vi "v4.0.vi"() -> ()   [LabVIEW 2018]
uses:
  <vilib>/DAQmx/read.llb/DAQmx Read (Analog 1D DBL NChan 1Samp).vi
  <extravilib>/ChannelInstances/High Speed Stream-c(a[.](c(dbl,dbl,dbl,dbl)),stamp,a[.](dbl),c(dbl,dbl,dbl,dbl,dbl,dbl,dbl))/_Read For Replicate.vi
  <extravilib>/ChannelInstances/High Speed Stream-c(a[.](c(dbl,dbl,dbl,dbl)),stamp,a[.](dbl),c(dbl,dbl,dbl,dbl,dbl,dbl,dbl))/Instantiate.vi
  <extravilib>/ChannelInstances/High Speed Stream-c(a[.](c(dbl,dbl,dbl,dbl)),stamp,a[.](dbl),c(dbl,dbl,dbl,dbl,dbl,dbl,dbl))/)Channel.vi
  <extravilib>/ChannelInstances/High Speed Stream-c(a[.](c(dbl,dbl,dbl,dbl)),stamp,a[.](dbl),c(dbl,dbl,dbl,dbl,dbl,dbl,dbl))/Abort Signal/Init Signal.vi
  <vilib>/Utility/file.llb/Write Delimited Spreadsheet (string).vi
  <vilib>/DAQmx/create/channels.llb/DAQmx Create Channel (AI-Temperature-Thermocouple).vi
  <vilib>/DAQmx/configure/timing.llb/DAQmx Timing (Sample Clock).vi
  <vilib>/DAQmx/miscellaneous.llb/DAQmx Fill In Error Info.vi
  <extravilib>/ChannelInstances/High Speed Stream-c(a[.](c(dbl,dbl,dbl,dbl)),stamp,a[.](dbl),c(dbl,dbl,dbl,dbl,dbl,dbl,dbl)).lvlib
  <resource>/objmgr/daqmx.rc
panel:
  out "SampClk.Rate":dbl
  out "Current Time":timestamp
  out "DAQmx Data":T1
  out "Rig Temperatures":T2
  out "Flowrate Data":T3(array[cluster])
  out "UI Current Time":timestamp format="%<%X\n%x>T"
  out "DAQ Current Time":timestamp format="%<%X\n%x>T"
  in  "file path (dialog if empty)":path
  out "Enum":T4(ring)
  in  "Start Recording?":bool
  in  "Stop Recording?":bool
  in  "Flowrate Control":dbl
  out "Status":T5(ring)
  in  "OK Button":bool
  in  "DAQ Properties":cluster{"Sample Rate [Hz]":dbl}={"Sample Rate [Hz]"=1.0} {"Sample Rate [Hz]" min=0.1 max=10000.0 step=0.1}
  # "Line Data [ °C]"
  # "Rig Temperatures [ °C]"
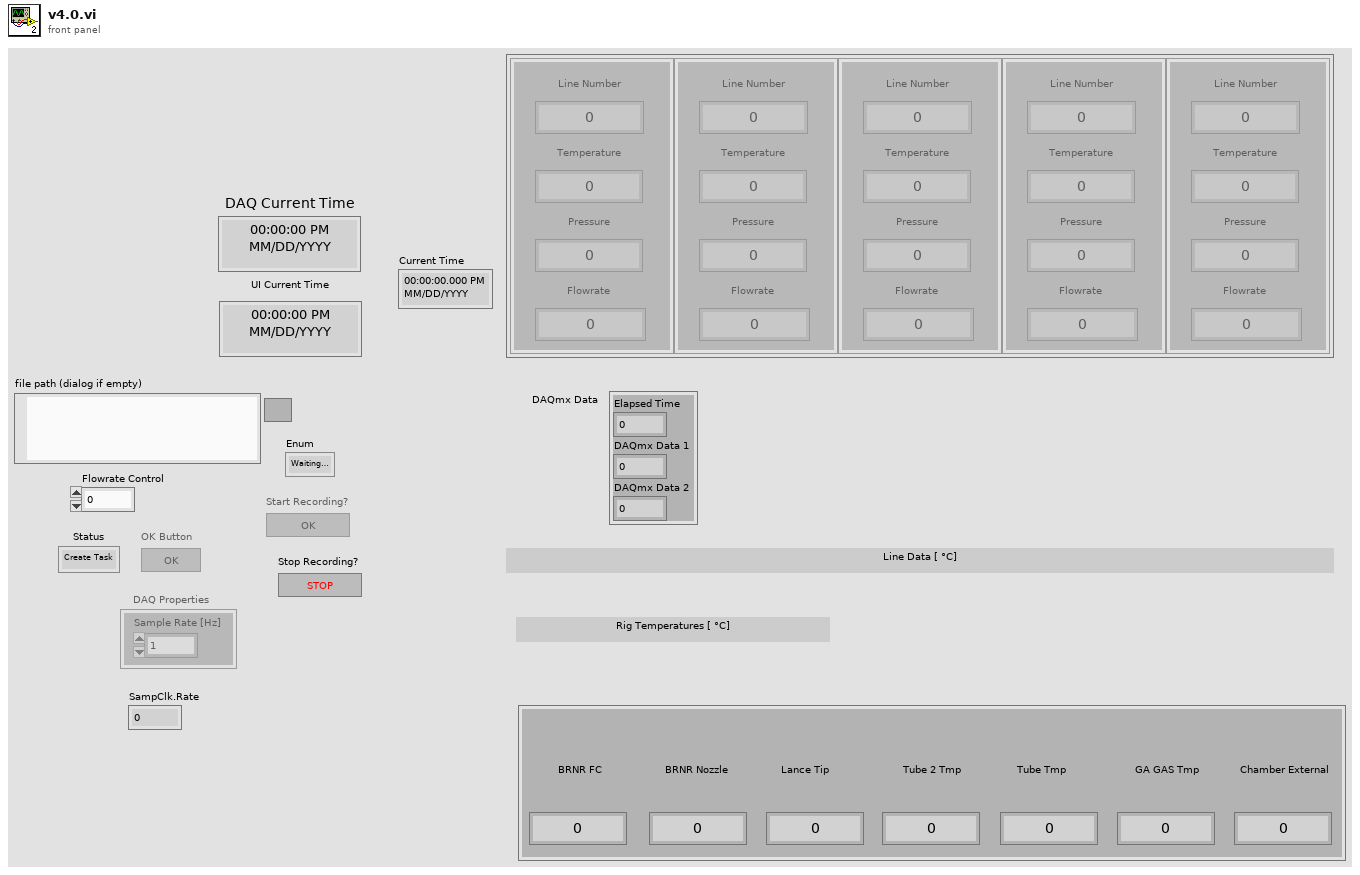
[diagram p1: front panel]
types:
  T1 = cluster{"Elapsed Time":dbl, "DAQmx Data 1":dbl, "DAQmx Data 2":dbl}
  T2 = cluster{"BRNR FC":dbl, "BRNR Nozzle":dbl, "Lance Tip":dbl, "Tube 2 Tmp":dbl, "Tube Tmp":dbl, "GA GAS Tmp":dbl, "Chamber External":dbl}
  T3 = cluster{"Line Number":dbl, "Temperature":dbl, "Pressure":dbl, "Flowrate":dbl}[]
  T4 = enum16{"Waiting to record", "Creating Spreadsheet", "Recording", "Finished Recording"}
  T5 = enum16{"Create Task", "Change Settings", "Check Settings", "Read Data", "End Task"}
  T6 = enum8{"Enabled", "Disabled", "Disabled and Grayed Out"}
  T7 = cluster{"Flowrate Data":cluster{"Line Number":dbl, "Temperature":dbl, "Pressure":dbl, "Flowrate":dbl}[], "Current Time":timestamp, "DAQmx Data":dbl[], "Rig Temperatures":cluster{"BRNR FC":dbl, "BRNR Nozzle":dbl, "Lance Tip":dbl, "Tube 2 Tmp":dbl, "Tube Tmp":dbl, "GA GAS Tmp":dbl, "Chamber External Temp":dbl}}
  T8 = cluster{"BRNR FC":dbl, "BRNR Nozzle":dbl, "Lance Tip":dbl, "Tube 2 Tmp":dbl, "Tube Tmp":dbl, "GA GAS Tmp":dbl, "Chamber External Temp":dbl}
  T9 = typedef "High Speed Stream-c(a[.](c(dbl,dbl,dbl,dbl)),stamp,a[.](dbl),c(dbl,dbl,dbl,dbl,dbl,dbl,dbl)).lvlib/)Channel.ctl" = refnum<queue>
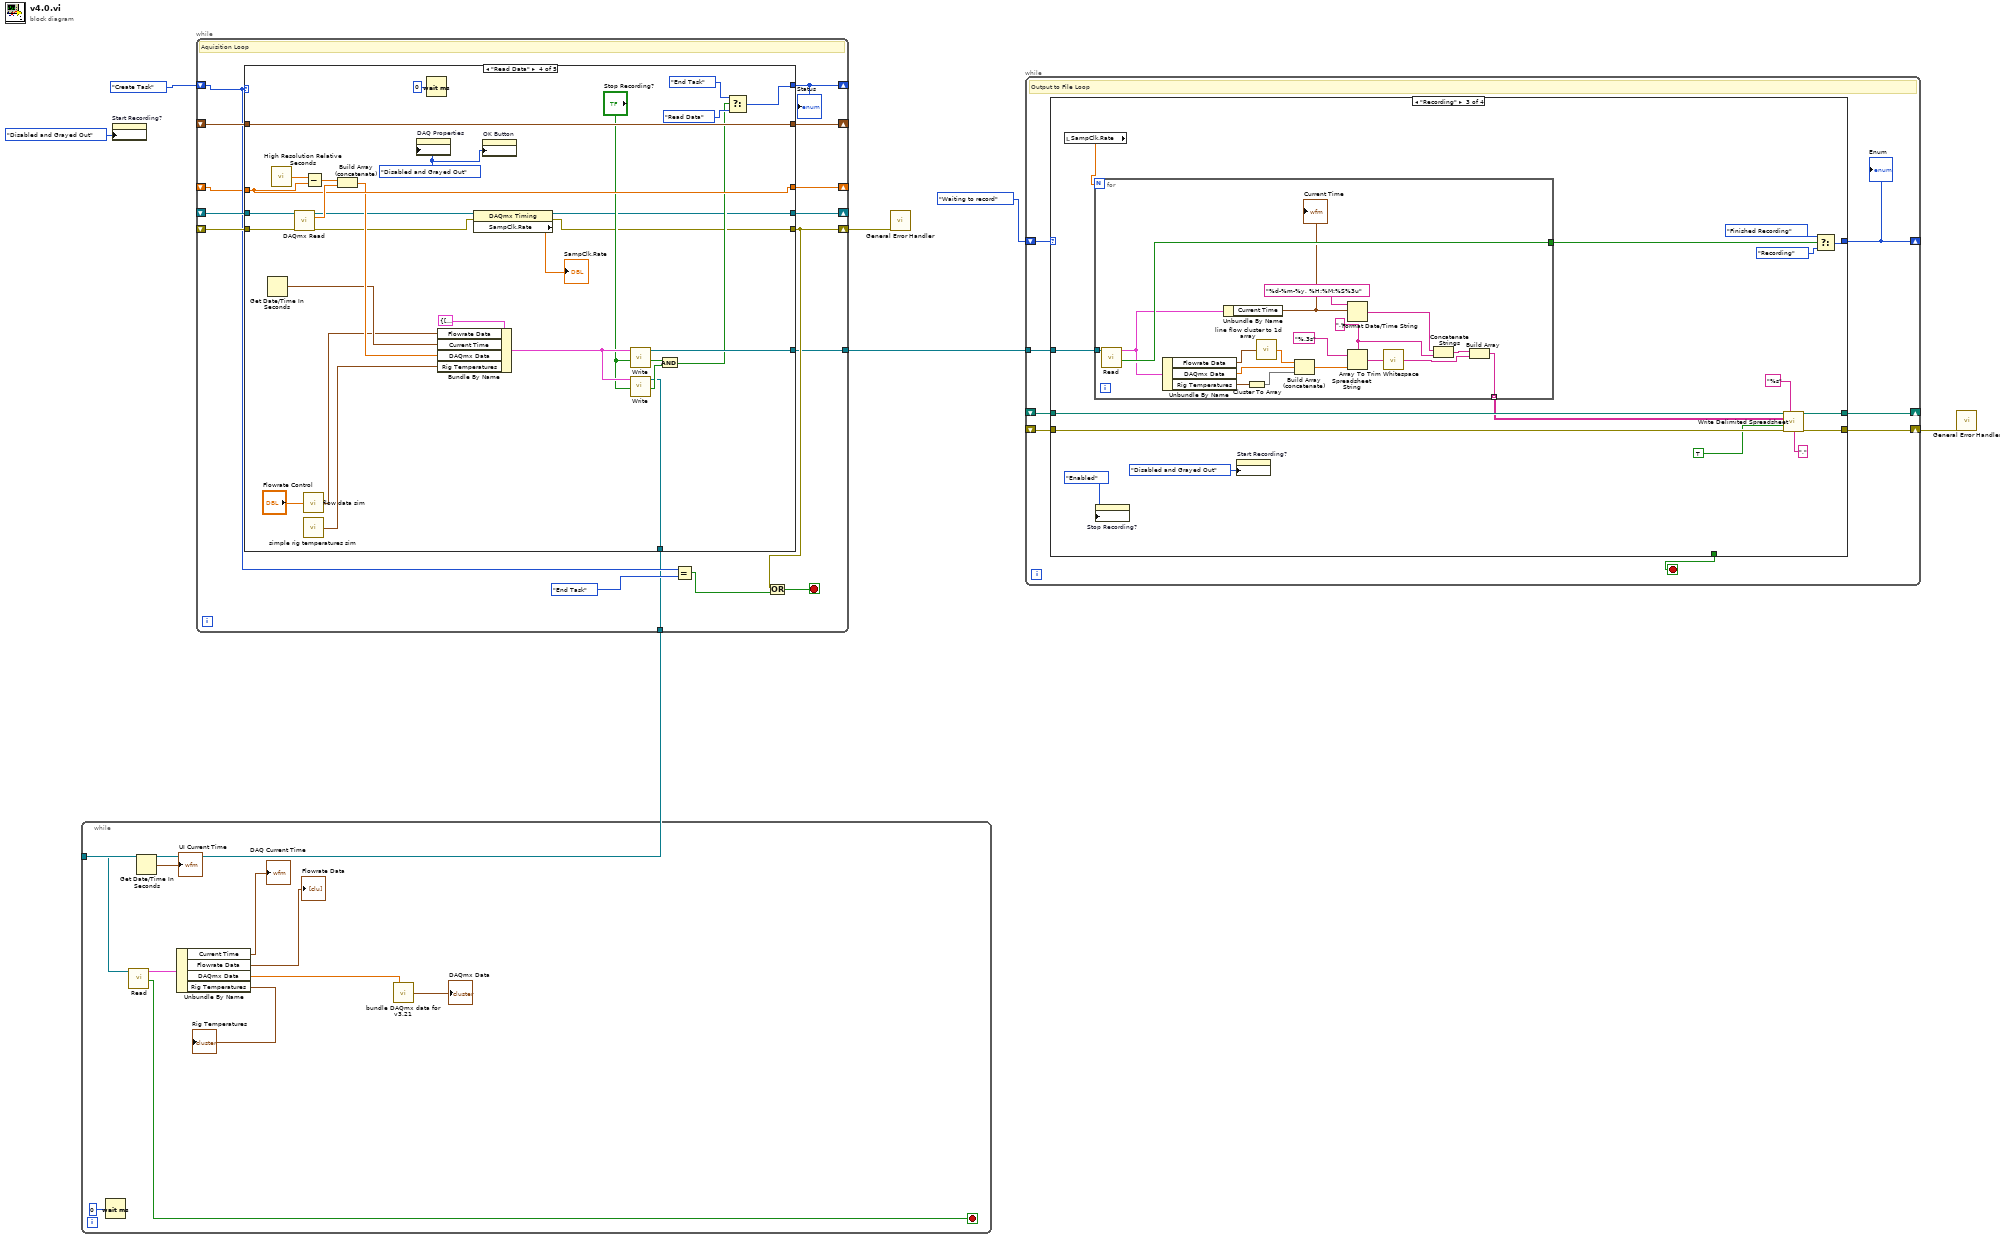
[diagram p0: block diagram]
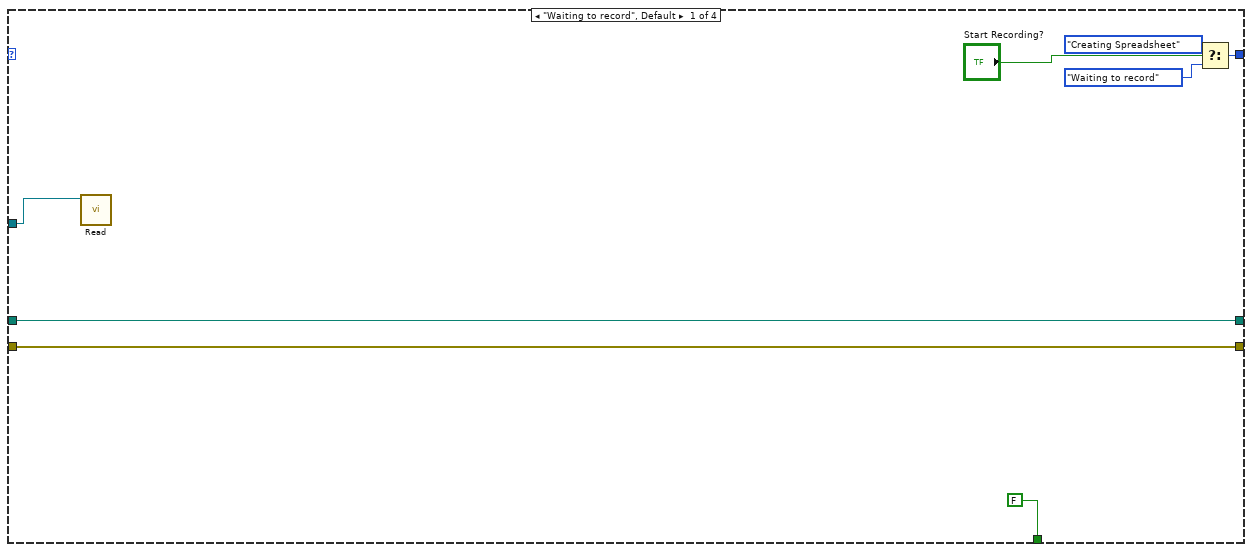
[diagram p2: hidden frame]
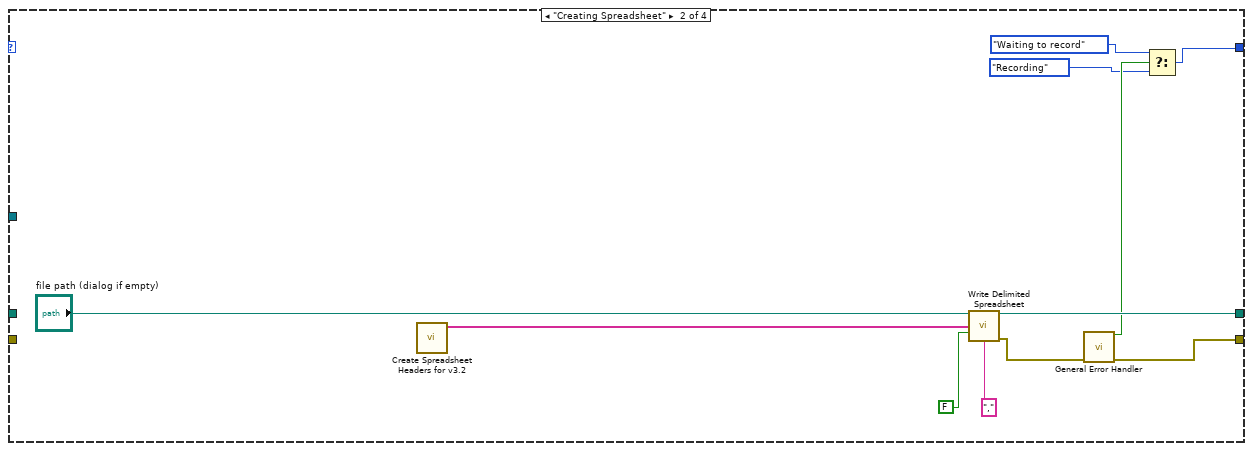
[diagram p3: hidden frame]
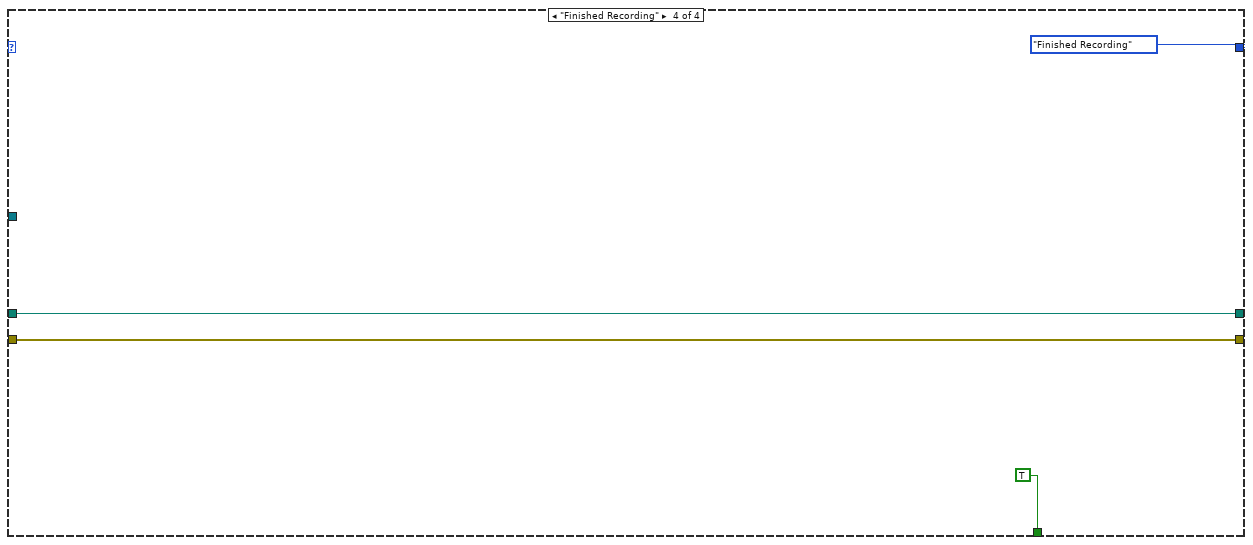
[diagram p4: hidden frame]
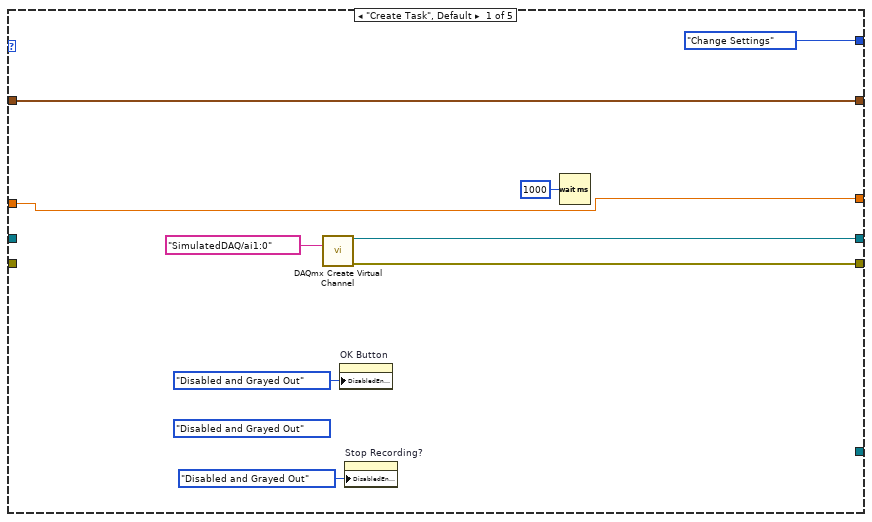
[diagram p5: hidden frame]
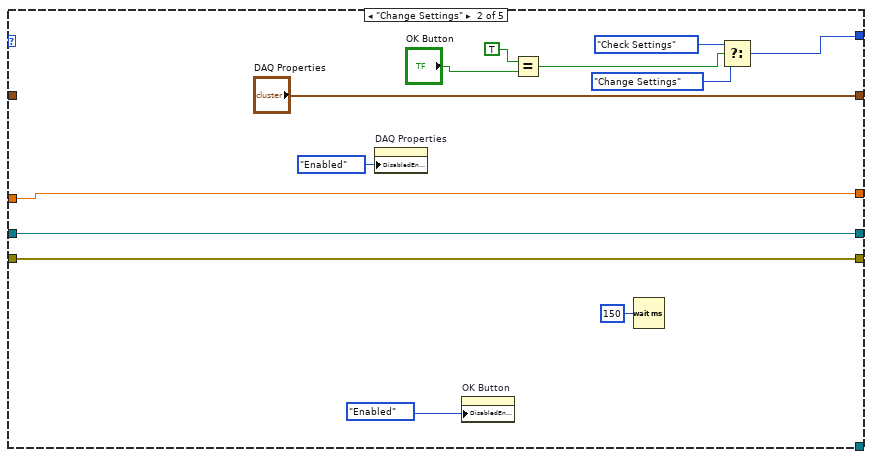
[diagram p6: hidden frame]
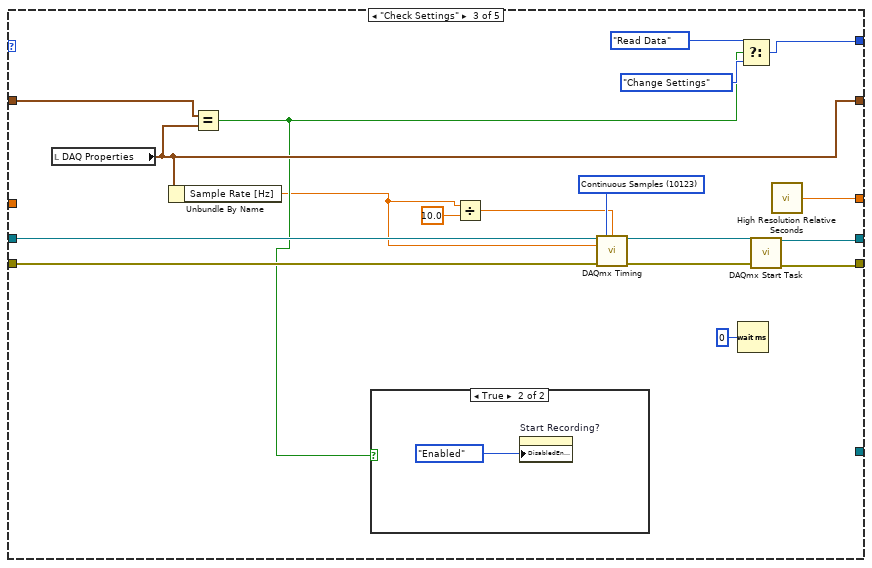
[diagram p7: hidden frame]
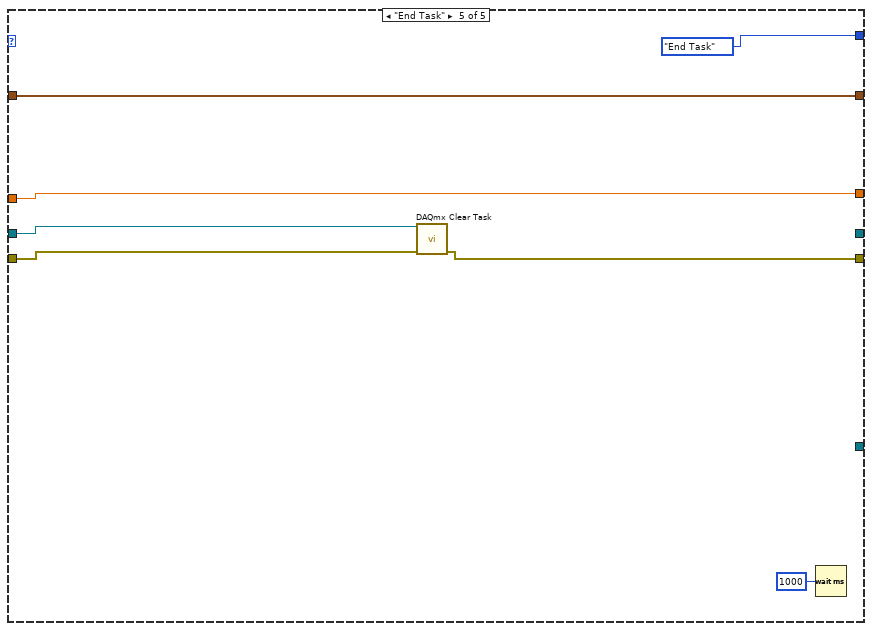
[diagram p9: hidden frame]
diagram:
  n1 = property on="Start Recording?" class="Bool"("DisabledEnum"=T6."Disabled and Grayed Out" ("Disabled")) -> ()  [unwired: 2 in, 2 out]
  n2 = while {
    shift-right: [w17] -> _
    shift-left: T5."Create Task" -> [w13]
    shift-right: [w22] -> _
    shift-left: _ -> [w20]
    shift-right: [w16] -> w3
    shift-left: _ -> [w19]
    shift-right: [w21] -> _
    shift-left: _ -> [w18]
    shift-right: [w12] -> _
    shift-left: _ -> [w11]
    tunnel: [w9] -> w5
    tunnel: [w8] -> w1
    stop <- w10 stop-if-true
    # "Aquisition Loop"
    n3 = case shown="\"Read Data\"" w13 {
      tunnel: [w31 w44 w52 w66 _] -> w22
      tunnel: [w30 w43 w51 w67 w100] -> w16
      tunnel: [T5."Change Settings" w37 w58 w89 T5."End Task"] -> w17
      tunnel: [w27 "DAQ Properties" w55 w91 w99] -> w21
      tunnel: w20 -> [_ w44 w57 w93 w97]
      tunnel: w19 -> [_ w43 w56 w92 w96]
      tunnel: w18 -> [w27 _ w62 w91 w99]
      tunnel: [w25 w34 w49 w83 w95] -> w12
      tunnel: w11 -> [w25 w34 _ w83 w95]
      tunnel: [_ _ _ w76 _] -> w9
      tunnel: [_ _ _ w69 _] -> w8
      frame "Create Task", Default {
        (unwired) T6."Disabled and Grayed Out" ("Disabled")
        n4 = call-poly <vilib>:"DAQmx Create Virtual Channel.vi"("physical channels"=tag "SimulatedDAQ/ai1:0") -> ("task out"=w31:refnum<k21>, "error out"=w30:errorcluster)  [unwired: 13 in]
        n5 = property on="OK Button" class="Bool"("DisabledEnum"=T6."Disabled and Grayed Out" ("Disabled")) -> ()  [unwired: 2 in, 2 out]
        n6 = property on="Stop Recording?" class="Bool"("DisabledEnum"=T6."Disabled and Grayed Out" ("Disabled")) -> ()  [unwired: 2 in, 2 out]
        n7 = Wait (ms)(milliseconds to wait=u32 1000) -> ()  [unwired: 1 out]
      }
      frame "Change Settings" {
        n8 = property on="DAQ Properties" class="Clust (strict)"("DisabledEnum"=T6."Enabled" ("Disabled")) -> ()  [unwired: 2 in, 2 out]
        n9 = property on="OK Button" class="Bool"("DisabledEnum"=T6."Enabled" ("Disabled")) -> ()  [unwired: 2 in, 2 out]
        n10 = Equal?(x=TRUE, y="OK Button") -> (x = y?=w39:bool)
        n11 = Wait (ms)(milliseconds to wait=u32 150) -> ()  [unwired: 1 out]
        n12 = Select(t=T5."Check Settings", s=w39, f=T5."Change Settings") -> (s? t:f=w37:T5)
      }
      frame "Check Settings" {
        w50 = 10123 items=["Finite Samples"=10178, "Continuous Samples"=10123, "Hardware Timed Single Point"=12522] ("sample mode")
        n13 = local read "DAQ Properties"() -> (w55:cluster{"Sample Rate [Hz]":dbl})
        n14 = Unbundle By Name(w55) -> ("Sample Rate [Hz]"=w46:dbl)
        n15 = Equal?(x=w62, y=w55) -> (x = y?=w48:bool)
        n16 = case shown="True" w48 {
          frame False {
          }
          frame True {
            n17 = property on="Start Recording?" class="Bool"("DisabledEnum"=T6."Enabled" ("Disabled")) -> ()  [unwired: 2 in, 2 out]
          }
        }
        n18 = Divide(x=w46, y=10.0) -> (x/y=w45:dbl)
        n19 = call-poly <vilib>:"DAQmx Timing.vi"("task/channels in"=w57, "sample mode"=w50, "samples per channel"=w45, "rate"=w46, "error in"=w56) -> ("task out"=w54:refnum<k21>, "error out"=w53:errorcluster)  [unwired: 9 in]
        n20 = Wait (ms)(milliseconds to wait=u32 0) -> ()  [unwired: 1 out]
        n21 = Select(t=T5."Read Data", s=w48, f=T5."Change Settings") -> (s? t:f=w58:T5)
        n22 = call <vilib>:"DAQmx Start Task.vi"("task/channels in"=w54, "error in"=w53) -> ("task out"=w52:refnum<k21>, "error out"=w51:errorcluster)  [unwired: 12 in]
        n23 = call <vilib>:"High Resolution Relative Seconds.vi"() -> ("relative seconds"=w49:dbl)
      }
      frame "Read Data" {
        w75 = T6."Disabled and Grayed Out" ("Disabled")
        n24 = Get Date/Time In Seconds() -> (seconds since 1Jan1904=w79:timestamp)
        n25 = call <vilib>:"High Resolution Relative Seconds.vi"() -> ("relative seconds"=w86:dbl)
        n26 = call-poly <vilib>:"DAQmx Read.vi"("task/channels in"=w93, "error in"=w92) -> ("task out"=w68:refnum<k21>, "data"=w85:dbl[], "error out"=w65:errorcluster)  [unwired: 11 in]
        n27 = call "simple rig temperatures sim.vi"() -> ("Rig Temperatures"=w77:T8)
        n28 = call "flow data sim.vi"("Offset"="Flowrate Control") -> ("Flowrate Data"=w78:T3)
        n29 = Subtract(x=w86, y=w83) -> (x-y=w84:dbl)
        n30 = Build Array (concatenate)(w84, w85) -> (w80:dbl[])
        n31 = property on="DAQ Properties" class="Clust (strict)"("DisabledEnum"=w75) -> ()  [unwired: 2 in, 2 out]
        n32 = Wait (ms)(milliseconds to wait=u32 0) -> ()  [unwired: 1 out]
        n33 = Bundle By Name(cluster=T7 {"Flowrate Data"=[{"Line Number"=1.0, "Temperature"=17.480721541683437, "Pressure"=24.0, "Flowrate"=0.0}, {"Line Number"=2.0, "Temperature"=21.850901927104296, "Pressure"=30.0, "Flowrate"=0.0}, {"Line Number"=3.0, "Temperature"=26.221082312525155, "Pressure"=36.0, "Flowrate"=0.0}, {"Line Number"=4.0, "Temperature"=30.591262697946018, "Pressure"=42.00000000000001, "Flowrate"=0.0}, {"Line Number"=5.0, "Temperature"=34.96144308336687, "Pressure"=48.0, "Flowrate"=0.0}], "Current Time"=timestamp(0 s since 1904-01-01), "DAQmx Data"=[], "Rig Temperatures"={"BRNR FC"=0.0, "BRNR Nozzle"=0.0, "Lance Tip"=0.0, "Tube 2 Tmp"=0.0, "Tube Tmp"=0.0, "GA GAS Tmp"=0.0, "Chamber External Temp"=0.0}}, "Flowrate Data"=w78, "Current Time"=w79, "DAQmx Data"=w80, "Rig Temperatures"=w77) -> (w74:T7)
        n34 = property class="DAQmx Timing"(reference=w68, error in=w65) -> (reference out=w66:refnum<k21>, error out=w67:errorcluster, "SampClk.Rate"=→"SampClk.Rate":dbl)
        n35 = property on="OK Button" class="Bool"("DisabledEnum"=w75) -> ()  [unwired: 2 in, 2 out]
        n36 = call <extravilib>:"Write.vi"("last element? (F)"="Stop Recording?", "element"=w74) -> ("done?"=w72:bool, "channel"=w76:T9)  [unwired: 7 in, 1 out]
        n37 = call <extravilib>:"Write.vi"("last element? (F)"="Stop Recording?", "element"=w74) -> ("done?"=w71:bool, "channel"=w69:T9)  [unwired: 7 in, 1 out]
        n38 = And(x=w72, y=w71) -> (x .and. y?=w70:bool)
        n39 = Select(t=T5."End Task", s=w70, f=T5."Read Data") -> (s? t:f=w89:T5)
      }
      frame "End Task" {
        n40 = call <vilib>:"DAQmx Clear Task.vi"("task in"=w97, "error in"=w96) -> ("error out"=w100:errorcluster)  [unwired: 13 in]
        n41 = Wait (ms)(milliseconds to wait=u32 1000) -> ()  [unwired: 1 out]
      }
    }
    "Status" <- w17
    n42 = Equal?(x=w13, y=T5."End Task") -> (x = y?=w14:bool)
    n43 = Or(x=w16, y=w14) -> (x .or. y?=w10:bool)
  }
  n44 = while {
    tunnel: w1 -> [w110]
    stop <- w109 stop-if-true
    n45 = Wait (ms)(milliseconds to wait=u32 0) -> ()  [unwired: 1 out]
    n46 = call <extravilib>:"Read.vi"("channel"=w110) -> ("done?"=w109:bool, "element"=w107:T7)  [unwired: 6 in, 3 out]
    n47 = Get Date/Time In Seconds() -> (seconds since 1Jan1904=→"UI Current Time":timestamp)
    n48 = Unbundle By Name(w107) -> ("Current Time"=→"DAQ Current Time":timestamp, "Flowrate Data"=→"Flowrate Data":T3, "DAQmx Data"=w103:dbl[], "Rig Temperatures"=→"Rig Temperatures":T8)
    n49 = call "bundle DAQmx data for v3.21 .vi"("DAQmx Data"=w103) -> ("DAQmx Data"=→"DAQmx Data":T1)
  }
  n50 = call <vilib>:"General Error Handler.vi"("error in (no error)"=w3) -> ()  [unwired: 10 in, 5 out]
  n51 = while {
    shift-right: [w118] -> _
    shift-left: T4."Waiting to record" -> [w117]
    tunnel: w5 -> [w115]
    shift-right: [w113] -> _
    shift-left: _ -> [w114]
    shift-right: [w112] -> w4
    shift-left: _ -> [w111]
    stop <- w116 stop-if-true
    # "Output to File Loop"
    n52 = case shown="\"Recording\"" w117 {
      tunnel: [w123 w129 w152 T4."Finished Recording"] -> w118
      tunnel: [FALSE _ _ TRUE] -> w116
      tunnel: w115 -> [w119 _ w149 _]
      tunnel: w114 -> [w121 _ w146 w173]
      tunnel: [w121 w137 w147 w173] -> w113
      tunnel: [w120 w131 w141 w172] -> w112
      tunnel: w111 -> [w120 _ w144 w172]
      frame "Waiting to record", Default {
        n53 = call <extravilib>:"Read.vi"("channel"=w119) -> ()  [unwired: 6 in, 5 out]
        n54 = Select(t=T4."Creating Spreadsheet", s="Start Recording?", f=T4."Waiting to record") -> (s? t:f=w123:T4)
      }
      frame "Creating Spreadsheet" {
        n55 = call "Create Spreadsheet Headers for v3.2.vi"() -> ("Array"=w136:string[])  [unwired: 11 in]
        n56 = call-poly <vilib>:"Write Delimited Spreadsheet.vi"("file path (dialog if empty)"="file path (dialog if empty)", "1D data"=w136, "append to file? (new file:F)"=FALSE, "delimiter (\\t)"="," ("delimiter (\\t)")) -> ("new file path (Not A Path if cancelled)"=w137:path, "error out"=w132:errorcluster)  [unwired: 10 in]
        n57 = call <vilib>:"General Error Handler.vi"("error in (no error)"=w132) -> ("error?"=w130:bool, "error out"=w131:errorcluster)  [unwired: 10 in, 3 out]
        n58 = Select(t=T4."Waiting to record", s=w130, f=T4."Recording") -> (s? t:f=w129:T4)
      }
      frame "Recording" {
        n59 = local read "SampClk.Rate"() -> (w138:dbl)
        n60 = for {
          N: w138 -> [_]
          tunnel: w149 -> [w170]
          tunnel: [w169] -> w148
          tunnel: [w154] -> w139 mode=indexing
          w159 = "," ("delimiter (Tab)")
          n61 = call <extravilib>:"Read.vi"("channel"=w170) -> ("done?"=w169:bool, "element"=w167:T7)  [unwired: 6 in, 3 out]
          n62 = Unbundle By Name(w167) -> ("Flowrate Data"=w168:T3, "DAQmx Data"=w165:dbl[], "Rig Temperatures"=w171:T8)
          n63 = Unbundle By Name(w167) -> ("Current Time"=w160:timestamp)
          "Current Time" <- w160
          n64 = Cluster To Array(cluster=w171) -> (array=w166:dbl[])
          n65 = call "line flow cluster to 1d array.vi"("Flowrate Data"=w168) -> ("Array"=w164:dbl[])
          n66 = Build Array (concatenate)(w164, w165, w166) -> (w157:dbl[])
          n67 = Format Date/Time String(time format string (%c)="%d-%m-%y, %H:%M:%S%3u", seconds (now)=w160) -> (date/time string=w158:string)  [unwired: 1 in]
          n68 = Array To Spreadsheet String(delimiter (Tab)=w159, array=w157, 3:"%.3s" ("format string")) -> (spreadsheet string=w163:string)
          n69 = call <vilib>:"Trim Whitespace.vi"("string"=w163) -> ("trimmed string"=w155:string)  [unwired: 1 in]
          n70 = Concatenate Strings(w158, w159) -> (w156:string)
          n71 = Build Array(w156, w155) -> (w154:string[])
        }
        n72 = property on="Stop Recording?" class="Bool"("DisabledEnum"=T6."Enabled" ("Disabled")) -> ()  [unwired: 2 in, 2 out]
        n73 = property on="Start Recording?" class="Bool"("DisabledEnum"=T6."Disabled and Grayed Out" ("Disabled")) -> ()  [unwired: 2 in, 2 out]
        n74 = call-poly <vilib>:"Write Delimited Spreadsheet.vi"("file path (dialog if empty)"=w146, "format (%s)"="%s", "2D data"=w139, "append to file? (new file:F)"=TRUE, "error in (no error)"=w144, "delimiter (\\t)"="," ("delimiter (\\t)")) -> ("new file path (Not A Path if cancelled)"=w147:path, "error out"=w141:errorcluster)  [unwired: 8 in]
        n75 = Select(t=T4."Finished Recording", s=w148, f=T4."Recording") -> (s? t:f=w152:T4)
      }
      frame "Finished Recording" {
      }
    }
    "Enum" <- w118
  }
  n76 = call <vilib>:"General Error Handler.vi"("error in (no error)"=w4) -> ()  [unwired: 10 in, 5 out]
